vi "PROJETO VF.vi"() -> ()   [LabVIEW 2018]
panel:
  out "Quantidade de Painéis Solares":i32
  in  "Média de horas de uso por dia 3":dbl format="%#_13g"
  in  "Média de horas de uso por dia 2":dbl format="%#_13g"
  in  "Média de horas de uso por dia":dbl format="%#_13g"
  out "Total  Gasto":dbl format="%#_13g"
  out "Total de Energia Gasto":dbl format="%#_13g"
  in  "Eletrodomésticos de       Baixo Consumo":dbl
  in  "Eletrodomésticos de       Alto Consumo":dbl
  in  "Eletrodomésticos de       Médio Consumo":dbl
  # "ENTRADAS:"
  # "RESULTADOS:"
  # "Manual de Instruções"
  # "Objetivo"
  # "É necessário que se indique, no bloco ENTRADAS, a quantidade de cada tipo de eletrodoméstico citado, tal como a média de horas por dia em que os eletrodomésticos são usados:\n1)Alto consumo (Fogão elétrico, aquecedores, chuveiros elétricos);\n2)Médio Consumo (ar condicionado, bombas d'água, lavadoura de louças), e\n3)Baixo Consumo (computadores, microondas, etc).\nFeito isso, o cliente terá como resultados a quantidade de energia gasta, o total gasto e a área da placa solar necessária para suprir essa quantidade de energia."
  # "O objetivo desse programa é mostrar quantos painéis solares o cliente necessitaria para suprir sua demanda de consumo de energia. \nPara isto, foi usado como exemplo um painel solar de 265 Watts de potência e com 80% de rendimento.\nA saída será o numero dos tais painéis necessários."
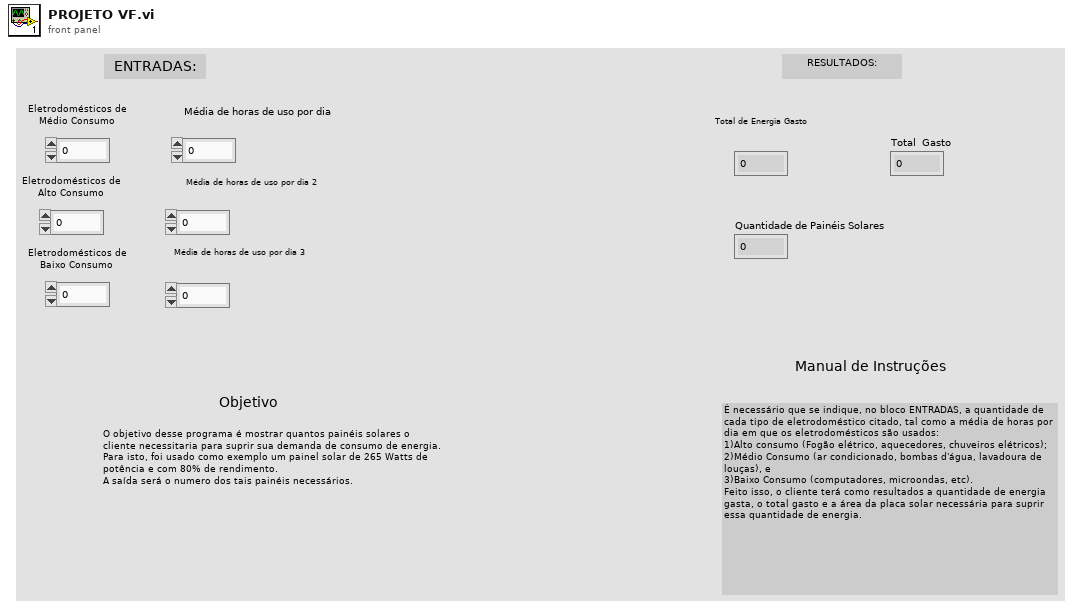
[diagram p1: front panel]
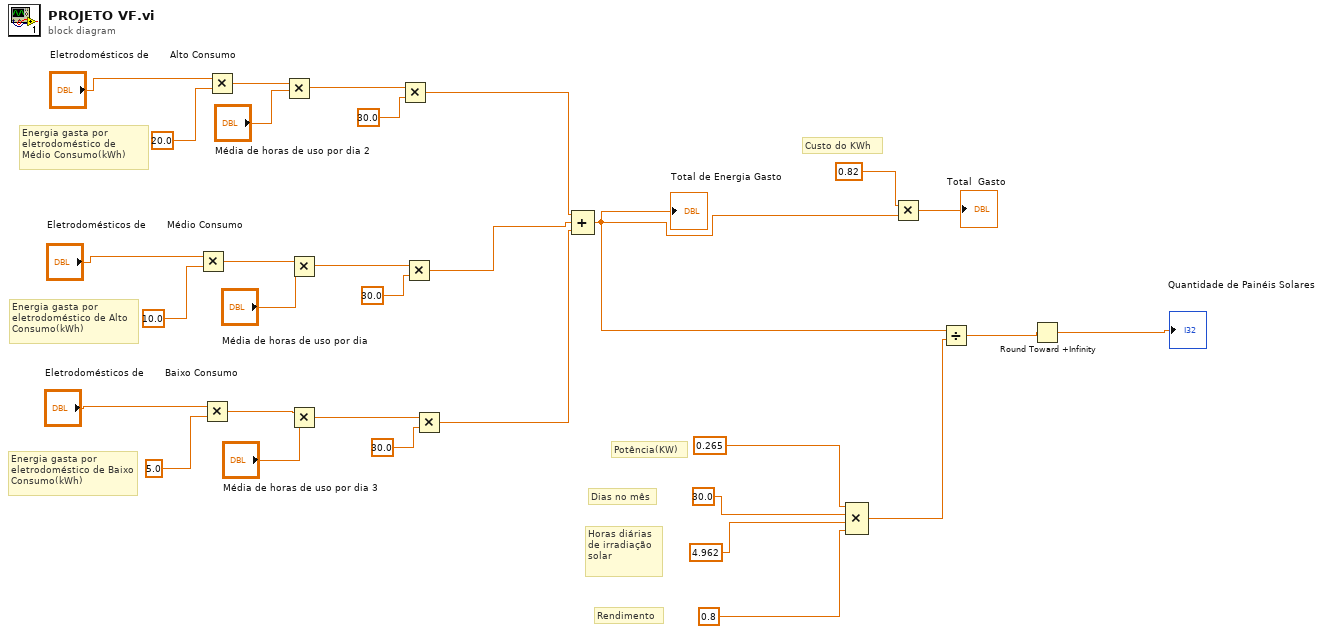
[diagram p0: block diagram]
diagram:
  # "Rendimento"
  # "Potência(KW)"
  # "Dias no mês"
  # "Horas diárias de irradiação solar"
  # "Custo do KWh"
  # "Energia gasta por eletrodoméstico de Baixo Consumo(kWh)"
  # "Energia gasta por eletrodoméstico de Alto Consumo(kWh)"
  # "Energia gasta por eletrodoméstico de Médio Consumo(kWh)"
  n1 = Multiply(x="Eletrodomésticos de       Médio Consumo", y=10.0) -> (x*y=w22:dbl)
  n2 = Multiply(x="Eletrodomésticos de       Baixo Consumo", y=5.0) -> (x*y=w21:dbl)
  n3 = Multiply(x="Eletrodomésticos de       Alto Consumo", y=20.0) -> (x*y=w23:dbl)
  n4 = Multiply(x=w23, y="Média de horas de uso por dia 2") -> (x*y=w19:dbl)
  n5 = Multiply(x=w22, y="Média de horas de uso por dia") -> (x*y=w16:dbl)
  n6 = Multiply(x=w21, y="Média de horas de uso por dia 3") -> (x*y=w14:dbl)
  n7 = Multiply(x=w19, y=30.0) -> (x*y=w18:dbl)
  n8 = Multiply(x=w16, y=30.0) -> (x*y=w12:dbl)
  n9 = Multiply(x=w14, y=30.0) -> (x*y=w13:dbl)
  n10 = Compound Arithmetic op=ADD(w18, w12, w13) -> (w5:dbl)
  "Total de Energia Gasto" <- w5
  n11 = Compound Arithmetic op=MULTIPLY(0.265, 30.0, 4.962, 0.8) -> (w6:dbl)
  n12 = Multiply(x=0.82, y=w5) -> (x*y=→"Total  Gasto":dbl)
  n13 = Divide(x=w5, y=w6) -> (x/y=w4:dbl)
  n14 = Round Toward +Infinity(x=w4) -> (ceil(x): smallest int >= x=→"Quantidade de Painéis Solares":dbl)
